vi "Update TC Temp CryoSep.vi"(8 "error in":errorcluster, 10 "TC Temperature":waveform(dbl)[](array[waveform]), 11 "Cryo Sep Results in":refnum<class "Cryo Sep Results.lvclass">) -> (0 "error out":errorcluster, 3 "Cryo Sep Results out":refnum<class "Cryo Sep Results.lvclass">)   [LabVIEW 2019, in "Results.lvlib" / "Cryo Sep Results.lvclass"]
uses:
  Cryo Sep Results.lvclass
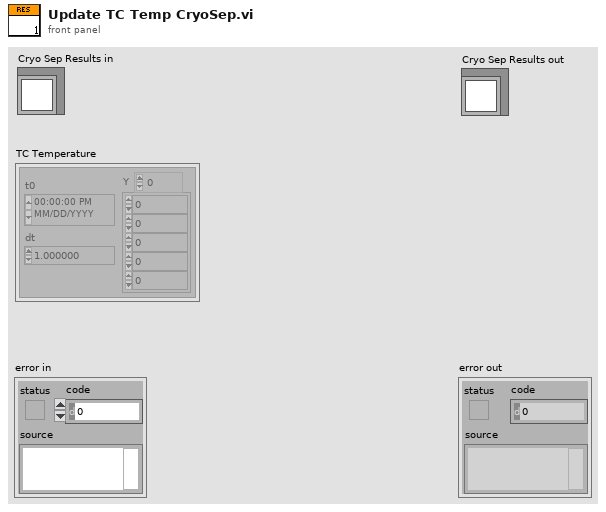
[diagram p1: front panel]
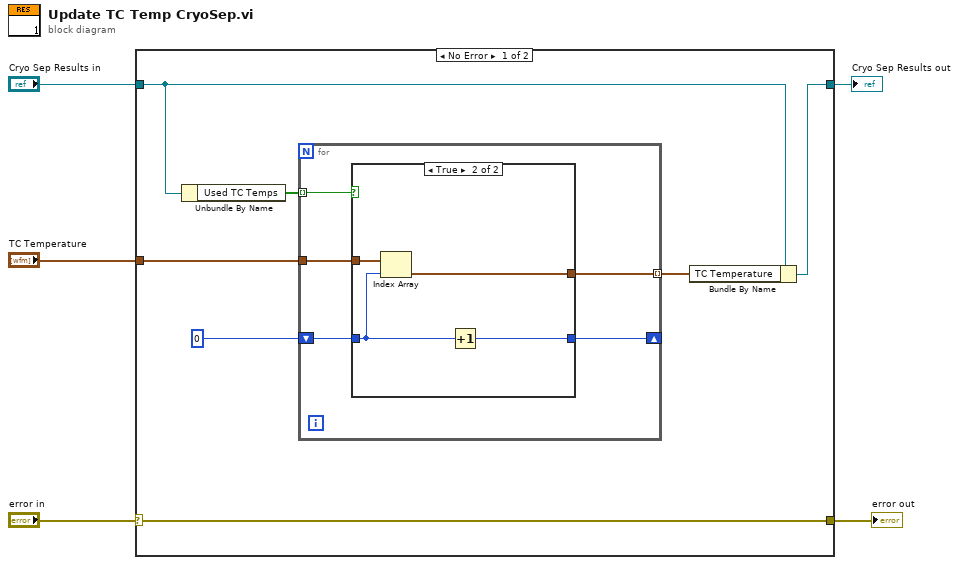
[diagram p0: block diagram]
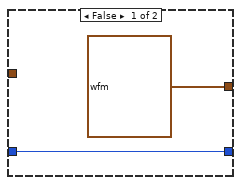
[diagram p2: hidden frame]
diagram:
  n1 = case shown="No Error" "error in" {
    selector: "error in" -> [w12 w24]
    tunnel: [w12 w24] -> w3
    tunnel: [w11 w25] -> w1
    tunnel: "Cryo Sep Results in" -> [w10 w25]
    tunnel: "TC Temperature" -> [w9 _]
    frame No Error {
      n2 = Unbundle By Name(w10) -> ("Used TC Temps"=w7:bool[])
      n3 = for {
        tunnel: w7 -> [w16] mode=indexing
        tunnel: w9 -> [w17]
        shift-right: [w14] -> _
        shift-left: 0 -> [w15]
        tunnel: [w13] -> w6 mode=indexing
        n4 = case shown="True" w16 {
          tunnel: w17 -> [_ w23]
          tunnel: w15 -> [w19 w22]
          tunnel: [w19 w21] -> w14
          tunnel: [waveform(dbl) {"t0"=timestamp(0 s since 1904-01-01), "dt"=1.0, "Y"=[]} ("element") w20] -> w13
          frame False {
          }
          frame True {
            n5 = Index Array(array=w23, index=w22) -> (element=w20:waveform(dbl))
            n6 = Increment(x=w22) -> (x+1=w21:i32)
          }
        }
      }
      n7 = Bundle By Name(cluster=w10, "TC Temperature"=w6) -> (w11:refnum<class "Cryo Sep Results.lvclass">)
    }
    frame Error {
    }
  }
  "error out" <- w3
  "Cryo Sep Results out" <- w1
